vi "read.vi"(8 "error in (no error)":errorcluster, 10 "timeout (ms)":i32=500, 11 "Tektronix RSA5106A in":refnum<class "Tektronix RSA5106A.lvclass">) -> (0 "error out":errorcluster, 2 "Return String":string, 3 "Tektronix RSA5106A out":refnum<class "Tektronix RSA5106A.lvclass">)   [LabVIEW 2013, in "Tektronix RSA5106A.lvclass"]
uses:
  Tektronix RSA5106A.lvclass
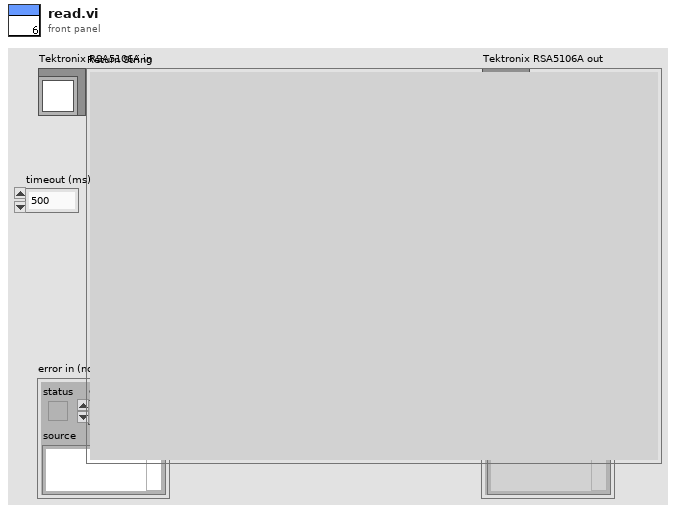
[diagram p1: front panel]
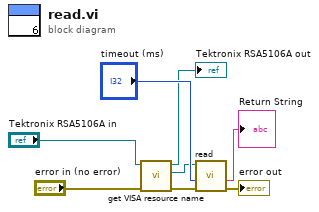
[diagram p0: block diagram]
diagram:
  n1 = call-dynamic "get VISA resource name.vi"("error in (no error)"="error in (no error)", "DeviceInterface (Eingang)"="Tektronix RSA5106A in") -> ("error out"=w5:errorcluster, "VISA resource name"=w4:refnum<visa-resource-name>, "DeviceInterface (Ausgang)"=→"Tektronix RSA5106A out":refnum<class "Tektronix RSA5106A.lvclass">)  [unwired: 7 in]
  n2 = call "read.vi"("error in (no error)"=w5, "timeout in ms"="timeout (ms)", "VISA resource name (COM Port of Prologix Device) in"=w4) -> ("error out"=→"error out":errorcluster, "output string"=→"Return String":string)  [unwired: 6 in, 1 out]
